vi "Klinger ConvUnitSgl.vi"(0 "ParamAct":dbl, 5 "UnitDem":u8(ring) caption="Unités\nDemandées" items=["Pas", "mm", "ps", "Degré (°)"], 7 "UnitAct":u8(ring)=2 caption="Unités\nActuelles" items=["Pas", "mm", "ps", "Degré (°)"], 9 "Axe":u8(ring)=3 items=["W", "X", "Y", "Z"], 11 "error in":errorcluster) -> (4 "ParamDem":dbl, 15 "error out":errorcluster)   [LabVIEW 2010]
doc: "Ce VI convertit le nombre spécifié de l'unitée actuelle vers l'unité demandée. Les différentes unité de déplacement disponible sont les pas, les µm et les picosecondes."
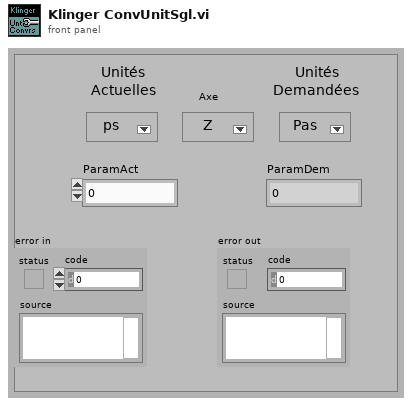
[diagram p1: front panel]
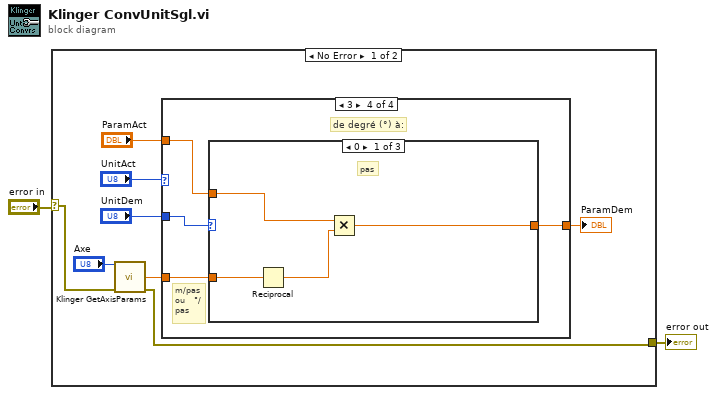
[diagram p0: block diagram]
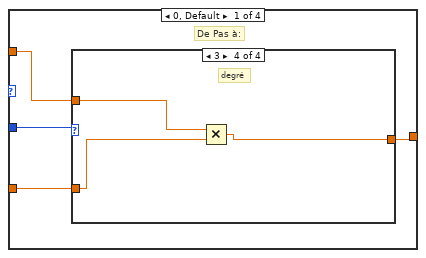
[diagram p2: hidden frame]
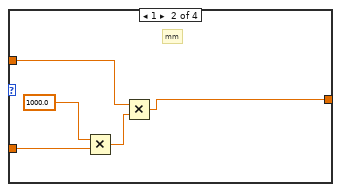
[diagram p4: hidden frame]
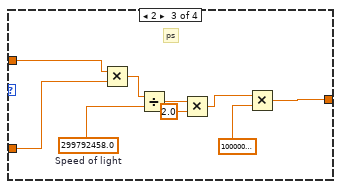
[diagram p5: hidden frame]
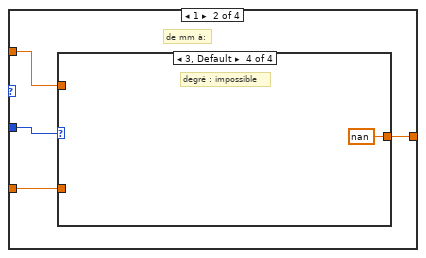
[diagram p6: hidden frame]
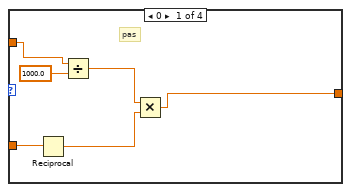
[diagram p7: hidden frame]
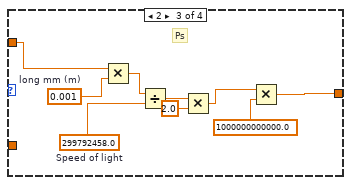
[diagram p9: hidden frame]
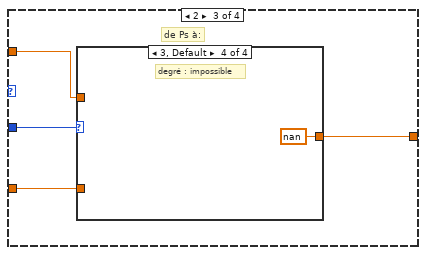
[diagram p10: hidden frame]
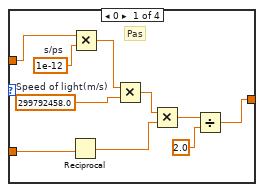
[diagram p11: hidden frame]
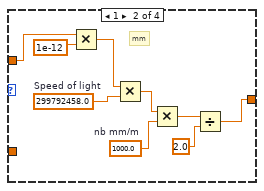
[diagram p12: hidden frame]
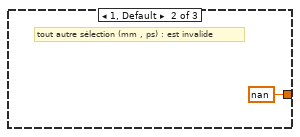
[diagram p14: hidden frame]
diagram:
  n1 = case shown="No Error" "error in" {
    selector: "error in" -> [w4 w89]
    tunnel: [w3 w89] -> w1
    frame No Error {
      n2 = call <userlib>:"Klinger GetAxisParams.vi"("Axe"="Axe", "error in"=w4) -> ("FactConv"=w6:dbl, "error out"=w3:errorcluster)  [unwired: 6 in, 6 out]
      n3 = case shown="3" "UnitAct" {
        tunnel: "UnitDem" -> [w12 w34 w57 w82]
        tunnel: "ParamAct" -> [w13 w36 w56 w81]
        tunnel: [w14 w35 w55 w80] -> w9
        tunnel: w6 -> [w11 w33 w54 w79]
        frame 0, Default {
          # "De Pas à:"
          n4 = case shown="3" w12 {
            tunnel: w13 -> [w15 w20 w25 w32]
            tunnel: [w15 w19 w23 w30] -> w14
            tunnel: w11 -> [_ w16 w21 w31]
            frame 0, Default {
              # "Pas"
            }
            frame 1 {
              # "mm"
              n5 = Multiply(x=1000.0, y=w16) -> (x*y=w17:dbl)
              n6 = Multiply(x=w20, y=w17) -> (x*y=w19:dbl)
            }
            frame 2 {
              w29 = 299792458.0  # Speed of light
              # "ps"
              n7 = Multiply(x=w25, y=w21) -> (x*y=w26:dbl)
              n8 = Divide(x=w26, y=w29) -> (x/y=w28:dbl)
              n9 = Multiply(x=w28, y=2.0) -> (x*y=w24:dbl)
              n10 = Multiply(x=w24, y=1000000000000.0) -> (x*y=w23:dbl)
            }
            frame 3 {
              # "degré"
              n11 = Multiply(x=w32, y=w31) -> (x*y=w30:dbl)
            }
          }
        }
        frame 1 {
          # "de mm à:"
          n12 = case shown="3, Default" w34 {
            tunnel: w36 -> [w39 w43 w47 _]
            tunnel: [w42 w43 w45 nan ("ParamAct")] -> w35
            tunnel: w33 -> [w40 _ _ _]
            frame 0 {
              # "pas"
              n13 = Reciprocal(x=w40) -> (1/x=w41:dbl)
              n14 = Divide(x=w39, y=1000.0) -> (x/y=w37:dbl)
              n15 = Multiply(x=w37, y=w41) -> (x*y=w42:dbl)
            }
            frame 1 {
              # "mm"
            }
            frame 2 {
              w49 = 0.001  # long mm (m)
              w52 = 299792458.0  # Speed of light
              # "Ps"
              n16 = Multiply(x=w47, y=w49) -> (x*y=w48:dbl)
              n17 = Divide(x=w48, y=w52) -> (x/y=w51:dbl)
              n18 = Multiply(x=w51, y=2.0) -> (x*y=w46:dbl)
              n19 = Multiply(x=w46, y=1000000000000.0) -> (x*y=w45:dbl)
            }
            frame 3, Default {
              # "degré : impossible"
            }
          }
        }
        frame 2 {
          # "de Ps à:"
          n20 = case shown="3, Default" w57 {
            tunnel: w56 -> [w61 w69 w77 _]
            tunnel: [w60 w68 w77 nan ("ParamAct")] -> w55
            tunnel: w54 -> [w58 _ _ _]
            frame 0 {
              w63 = 1e-12  # s/ps
              w64 = 299792458.0  # Speed of light(m/s)
              # "Pas"
              n21 = Reciprocal(x=w58) -> (1/x=w59:dbl)
              n22 = Multiply(x=w61, y=w63) -> (x*y=w62:dbl)
              n23 = Multiply(x=w62, y=w64) -> (x*y=w65:dbl)
              n24 = Multiply(x=w65, y=w59) -> (x*y=w67:dbl)
              n25 = Divide(x=w67, y=2.0) -> (x/y=w60:dbl)
            }
            frame 1 {
              w72 = 1000.0  # nb mm/m
              w73 = 299792458.0  # Speed of light
              # "mm"
              n26 = Multiply(x=w69, y=1e-12) -> (x*y=w70:dbl)
              n27 = Multiply(x=w70, y=w73) -> (x*y=w74:dbl)
              n28 = Multiply(x=w74, y=w72) -> (x*y=w76:dbl)
              n29 = Divide(x=w76, y=2.0) -> (x/y=w68:dbl)
            }
            frame 2 {
              # "Ps"
            }
            frame 3, Default {
              # "degré : impossible"
            }
          }
        }
        frame 3 {
          # "m/pas ou   °/pas"
          # "de degré (°) à:"
          n30 = case shown="0" w82 {
            tunnel: w81 -> [w84 _ w88]
            tunnel: [w83 nan ("ParamAct") w88] -> w80
            tunnel: w79 -> [w86 _ _]
            frame 0 {
              # "pas"
              n31 = Reciprocal(x=w86) -> (1/x=w85:dbl)
              n32 = Multiply(x=w84, y=w85) -> (x*y=w83:dbl)
            }
            frame 1, Default {
              # "tout autre sélection (mm , ps) : est invalide"
            }
            frame 3 {
              # "degré"
            }
          }
        }
      }
      "ParamDem" <- w9
    }
    frame Error {
    }
  }
  "error out" <- w1
